vi "hmi.vi"() -> ()   [LabVIEW 2017]
doc: "Demonstrates how to write and receive CAN frames via the Network Interface on the same port. \n\nTo write and receive frames via the Network Interface:\n- select the CAN Network Interface (i.e. CAN0, CAN1, etc.)\n- select the Baud Rate\n- run the VI\n- press the write button to write frames to the can bus\n\nEnable RTR Button to send a Remote Transmission Request or to simply send an empty Frame to request an Answer Frame from a connected device.\n\nEnable Extended Button to write extended Identifier Format. This is done by setting the 30th bit to enable extended format with the driver."
uses:
  <vilib>/nican/nican.llb/ncNetAttr.ctl
panel:
  in  "Tab Control":enum32{"Program", "Settings"}(tab)
  out "ID":u16 format="%04x"
  in  "Device":enum16{"Device 1", "Device 2"}(ring)
  out "Heartbeat":u16 format="%04x"
  in  "binFile":path
  in  "shutdown":bool
  in  "Initialize DFU":bool
  in  "Program":bool
  out "DFU Ready":bool
  in  "interface":string(combo)="CAN0" caption="Interface"
  # "PRESS AND HOLD"
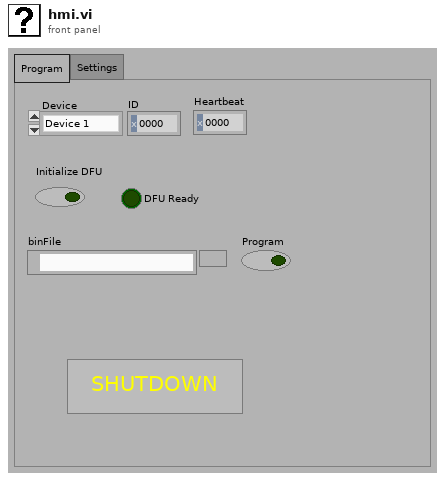
[diagram p1: front panel]
types:
  T1 = typedef "ncNetAttr.ctl" = cluster{"Start On Open":enum32{"FALSE", "TRUE"}, "Baud Rate":u32, "Read Queue Length":u32, "Write Queue Length":u32, "Standard Comparator":u32, "Standard Mask":u32, "Extended Comparator":u32, "Extended Mask":u32}
  T2 = typedef "xobjhandle.ctl" = u32
  T3 = typedef "CanFrameTimed.ctl" = cluster{"Timestamp":dbl, "ArbitrationId":u32, "IsRemote":u8, "DataLength":u8, "Data":u8[]}
  T4 = cluster{dbl, u32, "IsRemote":u8, "DataLength":u8, u8[]}
  T5 = cluster{dbl, u32, "IsRemote":u8, "DataLength":u8, u8[]}[]
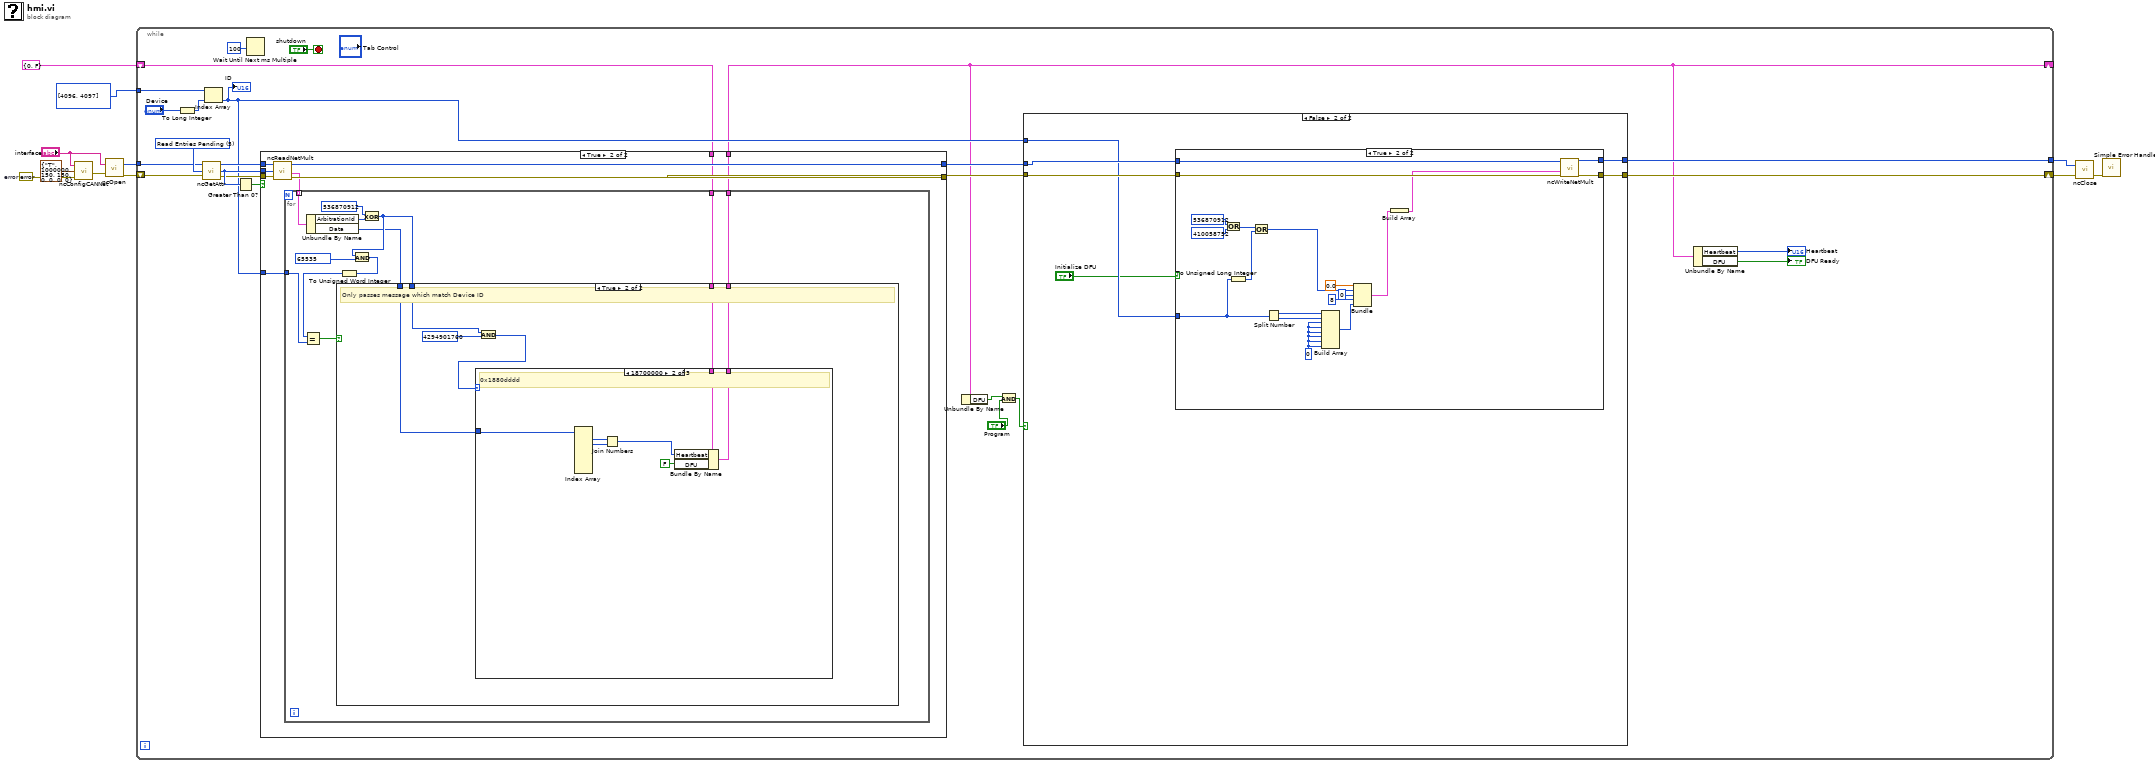
[diagram p0: block diagram]
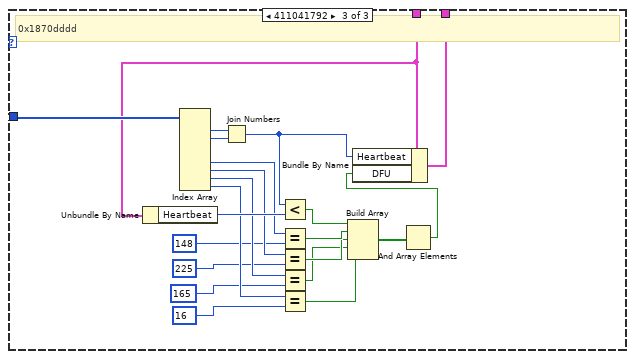
[diagram p5: hidden frame]
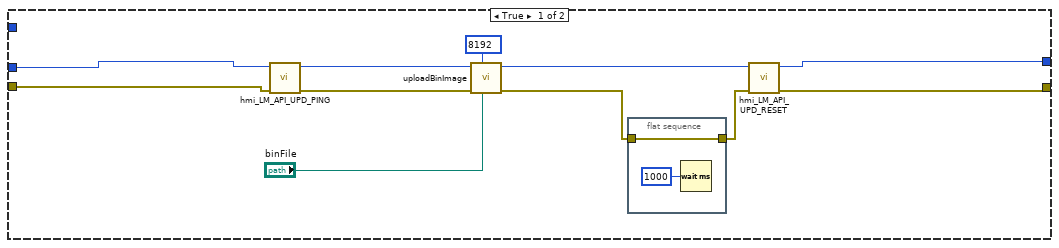
[diagram p6: hidden frame]
diagram:
  w7 = errorcluster {"status"=FALSE, "code"=0, "source"=""}  # error
  n1 = call <vilib>:"ncConfigCANNet.vi"("Error in"=w7, "CAN Network Interface Config"=T1 {"Start On Open"=enum."TRUE", "Baud Rate"=1000000, "Read Queue Length"=150, "Write Queue Length"=150, "Standard Comparator"=0, "Standard Mask"=0, "Extended Comparator"=0, "Extended Mask"=0}, "ObjName"="interface") -> ("Error out"=w8:errorcluster)  [unwired: 2 in]
  n2 = call <vilib>:"ncOpen.vi"("Error in"=w8, "ObjName"="interface") -> ("Error out"=w11:errorcluster, "ObjHandle out"=w9:T2)
  n3 = while {
    tunnel: w9 -> [w24]
    tunnel: [w34] -> w4
    shift-right: [w35] -> w3
    shift-left: w11 -> [w23]
    tunnel: u16[] [4096, 4097] -> [w22]
    shift-right: [w15] -> _
    shift-left: cluster{"Heartbeat":u16, "DFU":bool} {"Heartbeat"=0, "DFU"=FALSE} -> [w16]
    stop <- "shutdown" stop-if-true
    w27 = u32 5 items=["(reserved)", "Protocol Version", "Software Version", "Object State", "(reserved)", "Read Entries Pending", "Write Entries Pending", "ReadMult Size for Notification", "Listen Only?", "Self Reception?", "Transmit Error Counter", "Receive Error Counter", "Single Shot Transmit?", "Series 2 Filter Mode", "Series 2 Mask", "Series 2 Comparator", "Serial Number", "Form Factor", "Series", "Transceiver Type", "Interface Number", "Series 2 Error/Arb Capture", "Transceiver Mode", "Transceiver External Outputs", "Transceiver External Inputs", "Start Trigger Behavior", "Log Comm Warnings", "User RTSI Frame", "Transmit Mode", "Log Start Trigger?", "Timestamp Format", "Master Timebase Rate", "Virtual Bus Timing"] ("AttrId")
    n4 = To Long Integer(number="Device") -> (32bit integer=w20:i32)
    n5 = call <vilib>:"ncGetAttr.vi"("Error in"=w23, "AttrId"=w27, "ObjHandle in"=w24) -> ("Error out"=w28:errorcluster, "AttrValue"=w31:u32, "ObjHandle out"=w29:T2)
    n6 = Index Array(array=w22, index=w20) -> (element=w19:u16)
    "ID" <- w19
    n7 = Greater Than 0?(x=w31) -> (x > 0?=w30:bool)
    n8 = Wait Until Next ms Multiple(millisecond multiple=u32 100) -> ()  [unwired: 1 out]
    n9 = case shown="True" w30 {
      tunnel: [w37 w47] -> w25
      tunnel: [w38 w46] -> w26
      tunnel: w31 -> [_ w45]
      tunnel: w28 -> [w37 w44]
      tunnel: w29 -> [w38 w43]
      tunnel: w19 -> [_ w41]
      tunnel: w16 -> [w36 w40]
      tunnel: [w36 w39] -> w15
      frame False {
      }
      frame True {
        n10 = call <vilib>:"ncReadNetMult.vi"("ObjHandle in"=w43, "Requested Number of Frames"=w45, "Error in"=w44) -> ("ObjHandle out"=w46:T2, "Data"=w42:T3[], "Error out"=w47:errorcluster)  [unwired: 1 out]
        n11 = for {
          tunnel: w42 -> [w59] mode=indexing
          tunnel: w41 -> [w56]
          tunnel: w40 -> [w50]
          tunnel: [w49] -> w39
          n12 = Unbundle By Name(w59) -> ("ArbitrationId"=w57:u32, "Data"=w52:u8[])
          n13 = Exclusive Or(1:w57, 2:u32 536870912 ("y")) -> (0:w53:u32)
          n14 = And(x=w53, y=u32 65535) -> (x .and. y?=w55:u32)
          n15 = To Unsigned Word Integer(number=w55) -> (unsigned 16bit integer=w51:u16)
          n16 = Equal?(x=w51, y=w56) -> (x = y?=w54:bool)
          n17 = case shown="True" w54 {
            tunnel: w53 -> [_ w61]
            tunnel: w52 -> [_ w66]
            tunnel: w50 -> [w60 w64]
            tunnel: [w60 w63] -> w49
            frame False {
            }
            frame True {
              # "Only passes message which match Device ID"
              n18 = And(x=w61, y=u32 4294901760) -> (x .and. y?=w65:u32)
              n19 = case shown="18700000" w65 {
                tunnel: w66 -> [_ w72 w94]
                tunnel: w64 -> [w67 w71 w92]
                tunnel: [w67 w70 w93] -> w63
                frame Default {
                }
                frame 409993216 {
                  # "0x1880dddd"
                  n20 = Index Array(array=w72) -> (element #1=w73:u8, element #2=w74:u8)  [unwired: 8 in, 6 out]
                  n21 = Join Numbers(hi=w73, lo=w74) -> ((hi.lo)=w69:u16)
                  n22 = Bundle By Name(cluster=w71, "Heartbeat"=w69, "DFU"=FALSE) -> (w70:cluster{"Heartbeat":u16, "DFU":bool})
                }
                frame 411041792 {
                  # "0x1870dddd"
                  n23 = Unbundle By Name(w92) -> ("Heartbeat"=w91:u16)
                  n24 = Index Array(array=w94) -> (element #1=w95:u8, element #2=w96:u8, element #5=w84:u8, element #6=w83:u8, element #7=w82:u8, element #8=w81:u8)  [unwired: 8 in, 2 out]
                  n25 = Join Numbers(hi=w95, lo=w96) -> ((hi.lo)=w90:u16)
                  n26 = Less?(x=w90, y=w91) -> (x < y?=w89:bool)
                  n27 = Equal?(x=w84, y=u8 148) -> (x = y?=w88:bool)
                  n28 = Equal?(x=w83, y=u8 225) -> (x = y?=w87:bool)
                  n29 = Equal?(x=w82, y=u8 165) -> (x = y?=w86:bool)
                  n30 = Equal?(x=w81, y=u8 16) -> (x = y?=w85:bool)
                  n31 = Build Array(w89, w88, w87, w86, w85) -> (w76:bool[])
                  n32 = And Array Elements(Boolean array=w76) -> (logical AND=w75:bool)
                  n33 = Bundle By Name(cluster=w92, "Heartbeat"=w90, "DFU"=w75) -> (w93:cluster{"Heartbeat":u16, "DFU":bool})
                }
              }
            }
          }
        }
      }
    }
    n34 = Unbundle By Name(w15) -> ("DFU"=w12:bool)
    n35 = And(x=w12, y="Program") -> (x .and. y?=w13:bool)
    n36 = case shown="False" w13 {
      tunnel: [w97 w115] -> w35
      tunnel: [w98 w114] -> w34
      tunnel: w26 -> [w100 w113]
      tunnel: w25 -> [w99 w112]
      tunnel: w19 -> [_ w111]
      frame True {
        n37 = call "hmi_LM_API_UPD_PING.vi"("Error in"=w99, "canSession"=w100) -> ("Error out"=w105:errorcluster, "canSession"=w106:T2)  [unwired: 7 in, 1 out]
        n38 = call "uploadBinImage.vi"("binFile"="binFile", "dloadAddr"=u32 8192 ("dloadSize"), "Error in"=w105, "canSession"=w106) -> ("Error out"=w104:errorcluster, "canSession"=w103:T2)  [unwired: 5 in, 1 out]
        n39 = flat-sequence {
          tunnel: w104 -> [w109]
          tunnel: [w109] -> w107
          frame #0 {
            n40 = Wait (ms)(milliseconds to wait=u32 1000) -> ()  [unwired: 1 out]
          }
        }
        n41 = call "hmi_LM_API_UPD_RESET.vi"("Error in"=w107, "canSession"=w103) -> ("Error out"=w97:errorcluster, "canSession"=w98:T2)  [unwired: 8 in]
      }
      frame False {
        n42 = case shown="True" "Initialize DFU" {
          tunnel: [w116 w136] -> w115
          tunnel: [w117 w135] -> w114
          tunnel: w113 -> [w117 w134]
          tunnel: w112 -> [w116 w133]
          tunnel: w111 -> [_ w121]
          frame False {
          }
          frame True {
            w132 = u8 0
            n43 = Or(x=u32 536870912 ("y"), y=u32 410058752) -> (x .or. y?=w119:u32)
            n44 = To Unsigned Long Integer(number=w121) -> (unsigned 32bit integer=w120:u32)
            n45 = Or(x=w119, y=w120) -> (x .or. y?=w118:u32)
            n46 = Split Number(x=w121) -> (hi(x)=w125:u8, lo(x)=w124:u8)
            n47 = Build Array(w125, w124, w132, w132, w132, w132, w132, w132) -> (w130:u8[])
            n48 = Bundle(0.0, w118, "IsRemote"=u8 0, "DataLength"=u8 8, w130) -> (w123:T4)  [unwired: 1 in]
            n49 = Build Array(w123) -> (w122:T5)
            n50 = call <vilib>:"ncWriteNetMult.vi"("Error in"=w133, "Data"=w122, "ObjHandle in"=w134) -> ("Error out"=w136:errorcluster, "ObjHandle out"=w135:T2)  [unwired: 7 in]
          }
        }
      }
    }
    n51 = Unbundle By Name(w15) -> ("Heartbeat"=→"Heartbeat":u16, "DFU"=→"DFU Ready":bool)
  }
  n52 = call <vilib>:"ncClose.vi"("Error in"=w3, "ObjHandle in"=w4) -> ("Error out"=w5:errorcluster)  [unwired: 1 in]
  n53 = call <vilib>:"Simple Error Handler.vi"("error in (no error)"=w5) -> ()  [unwired: 4 in, 5 out]
